vi "Write Camera Setup.vi"(8 "error in (no error)":errorcluster, 10 "Camera Setup":T1={"Image Name"="Image", "Image Path"="C:\\Users\\Cliente\\Desktop\\SPARC4_AC\\Imagens\\", "#FRAMES"=0, "EXPTIME"=0.0, "PREAMP"=0, "READOUT_RATE"=0, "VERTICAL_SHIFT_SPEED"=3, "ACQUISITION_MODE"=1, "READ_MODE"=4, "EM_MODE"=0, "EM_GAIN"=2, "SHUTTER_MODE"=2, "SHUTTER_TTL"=0, "SHUTTER_OPENNING_TIME"=50, "SHUTTER_CLOSING_TIME"=50, "VBIN"=1, "HBIN"=1, "INITAIL_LINE"=1, "INITIAL_COLUMN"=1, "FINAL_LINE"=1024, "FINAL_COLUMN"=1024, "Cooler ON/OFF"=0, "Set temperature"=20, "Exposições realizadas"=0, "Kinetic Serie Length"=0, "Number of Accumulations"=0, "Kinetic Cycle Time"=0, "FRAME_TRANSFER"=FALSE, "VERTICAL_CLOCK_VOLTAGE"=0, "TRIGGER_MODE"=0, "Number of exp"=0, "AD_CHANNEL"=0} {"TRIGGER_MODE" items=["Internal", "External", "N/A", "N/A", "N/A", "N/A", "External Start"]; "VERTICAL_CLOCK_VOLTAGE" items=["Normal", "+1", "+2", "+3", "+4"]; "Set temperature" min=0 max=0; "Cooler ON/OFF" items=["Cooler OFF", "Cooler ON"]; "SHUTTER_TTL" items=["TTL Low", "TTl High"]; "SHUTTER_MODE" items=["Fully Auto", "OPEN", "CLOSED"]; "EM_MODE" items=["Electron Multiplying", "Conventional"]; "READ_MODE" items=["Full Vertical Binning", "Multi-Track", "Random-track", "Single-Track", "Image"]; "ACQUISITION_MODE" items=["N/A", "Single", "Accumulate", "Kinetic", "Fast Kinetic"]; "VERTICAL_SHIFT_SPEED" items=["0.6", "1.13", "2.2", "4.33"]; "READOUT_RATE" items=["1 MHz", "10 MHz", "20 MHz", "30 MHz"]; "PREAMP" items=["Gain 1", "Gain 2"]}, 11 "Interface in":refnum<class "Interface.lvclass">) -> (0 "error out":errorcluster, 3 "Interface out":refnum<class "Interface.lvclass">)   [LabVIEW 2018, in "Interface.lvclass"]
uses:
  Interface.lvclass
  Interface.lvclass/Interface.ctl
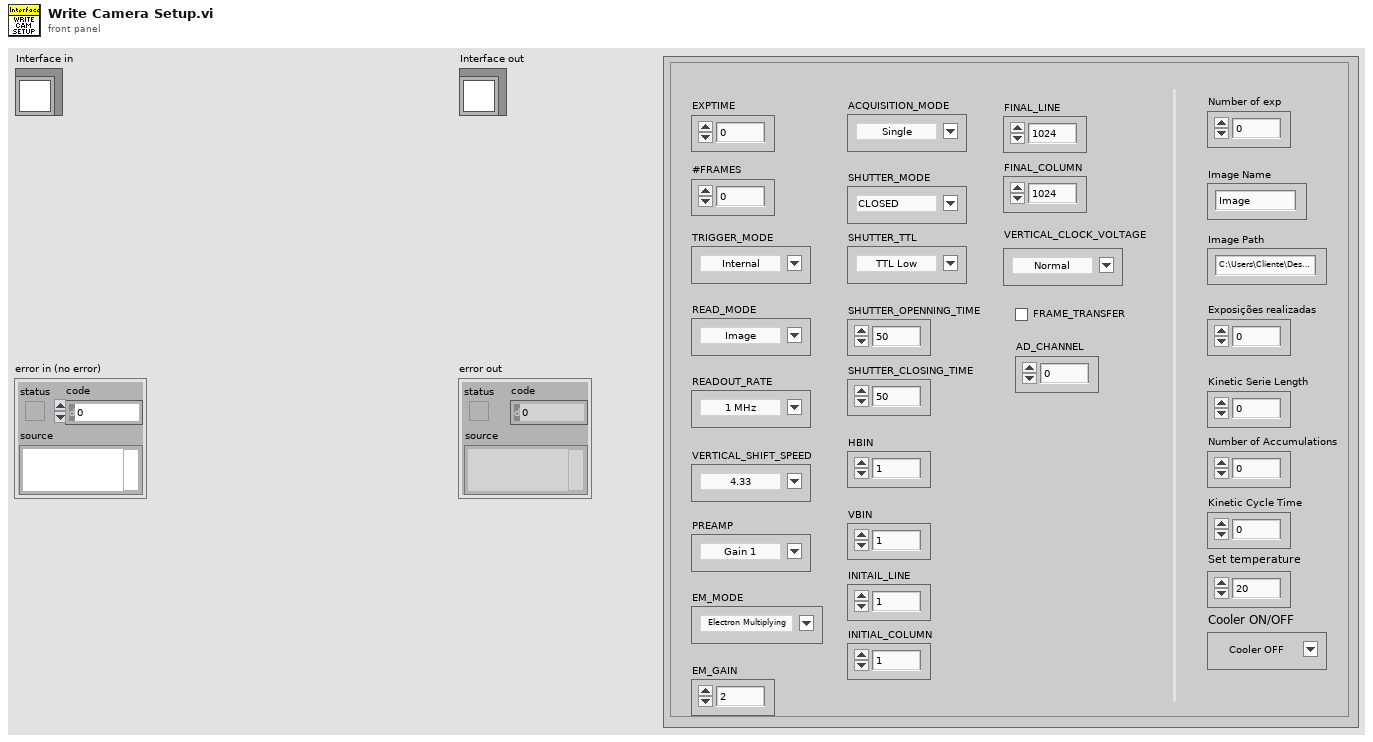
[diagram p1: front panel]
types:
  T1 = cluster{"Image Name":string, "Image Path":string, "#FRAMES":u32, "EXPTIME":dbl, "PREAMP":u8, "READOUT_RATE":u8, "VERTICAL_SHIFT_SPEED":u8, "ACQUISITION_MODE":u8, "READ_MODE":u8, "EM_MODE":u8, "EM_GAIN":u16, "SHUTTER_MODE":u8, "SHUTTER_TTL":u8, "SHUTTER_OPENNING_TIME":u16, "SHUTTER_CLOSING_TIME":u16, "VBIN":u16, "HBIN":u16, "INITAIL_LINE":u16, "INITIAL_COLUMN":u16, "FINAL_LINE":u16, "FINAL_COLUMN":u16, "Cooler ON/OFF":u16, "Set temperature":i8, "Exposições realizadas":u16, "Kinetic Serie Length":u32, "Number of Accumulations":u32, "Kinetic Cycle Time":u32, "FRAME_TRANSFER":bool, "VERTICAL_CLOCK_VOLTAGE":u8, "TRIGGER_MODE":u8, "Number of exp":u32, "AD_CHANNEL":u32}
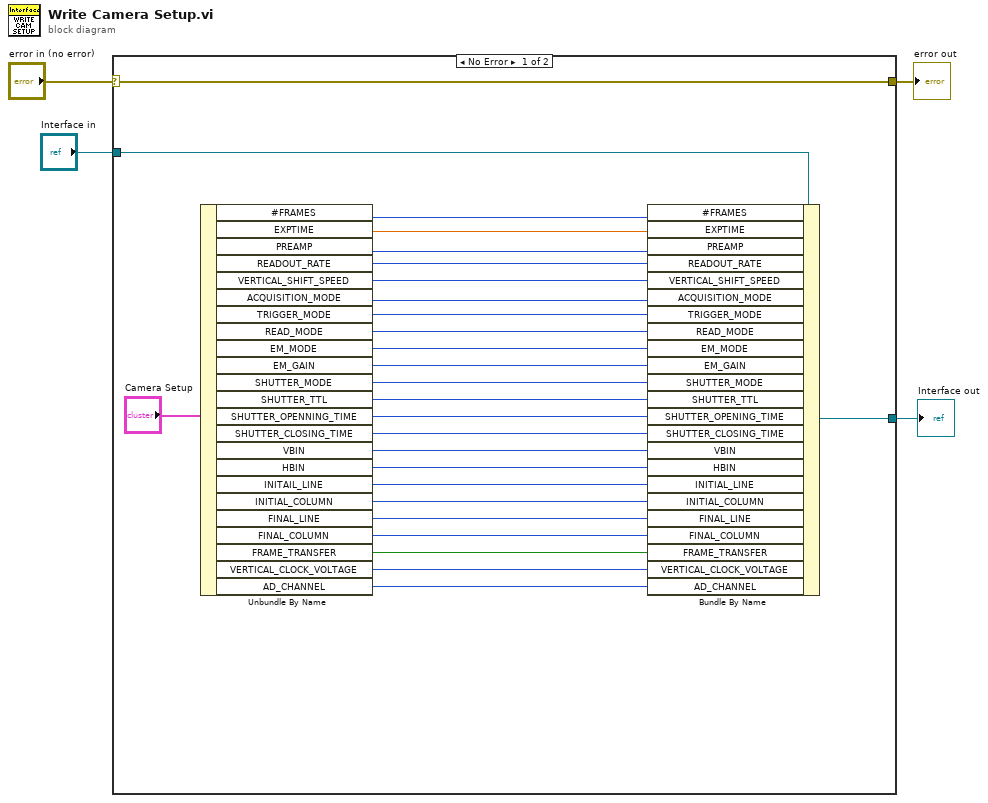
[diagram p0: block diagram]
diagram:
  n1 = case shown="No Error" "error in (no error)" {
    selector: "error in (no error)" -> [w31 w33]
    tunnel: [w31 w33] -> w3
    tunnel: [w9 w32] -> w1
    tunnel: "Interface in" -> [w30 w32]
    frame No Error {
      n2 = Unbundle By Name("Camera Setup") -> ("#FRAMES"=w10:u32, "EXPTIME"=w11:dbl, "PREAMP"=w12:u8, "READOUT_RATE"=w13:u8, "VERTICAL_SHIFT_SPEED"=w14:u8, "ACQUISITION_MODE"=w15:u8, "TRIGGER_MODE"=w16:u8, "READ_MODE"=w17:u8, "EM_MODE"=w18:u8, "EM_GAIN"=w19:u16, "SHUTTER_MODE"=w20:u8, "SHUTTER_TTL"=w21:u8, "SHUTTER_OPENNING_TIME"=w22:u16, "SHUTTER_CLOSING_TIME"=w23:u16, "VBIN"=w24:u16, "HBIN"=w25:u16, "INITAIL_LINE"=w26:u16, "INITIAL_COLUMN"=w27:u16, "FINAL_LINE"=w28:u16, "FINAL_COLUMN"=w29:u16, "FRAME_TRANSFER"=w7:bool, "VERTICAL_CLOCK_VOLTAGE"=w6:u8, "AD_CHANNEL"=w5:u32)
      n3 = Bundle By Name(cluster=w30, "#FRAMES"=w10, "EXPTIME"=w11, "PREAMP"=w12, "READOUT_RATE"=w13, "VERTICAL_SHIFT_SPEED"=w14, "ACQUISITION_MODE"=w15, "TRIGGER_MODE"=w16, "READ_MODE"=w17, "EM_MODE"=w18, "EM_GAIN"=w19, "SHUTTER_MODE"=w20, "SHUTTER_TTL"=w21, "SHUTTER_OPENING_TIME"=w22, "SHUTTER_CLOSING_TIME"=w23, "VBIN"=w24, "HBIN"=w25, "INITIAL_LINE"=w26, "INITIAL_COLUMN"=w27, "FINAL_LINE"=w28, "FINAL_COLUMN"=w29, "FRAME_TRANSFER"=w7, "VERTICAL_CLOCK_VOLTAGE"=w6, "AD_CHANNEL"=w5) -> (w9:refnum<class "Interface.lvclass">)
    }
    frame Error {
    }
  }
  "error out" <- w3
  "Interface out" <- w1
